vi "Reset Pin Names.vi"(0 "Display State In":T1, 7 "Connector":string="roboRIO 10 Bank Connector DIO", 9 "Container State":T2, 11 "error in (no error)":errorcluster) -> (4 "Display State Out":T1, 15 "error out":errorcluster)   [LabVIEW 2021, in "roboRIO 10 Bank.xctl"]
uses:
  <vilib>/myRIO/Common/Instrument Driver Framework/Utilities/xctls/roboRIO 10 Bank/roboRIO 10 Bank.xctl
  <vilib>/_xctls/Container State.ctl
  <vilib>/myRIO/Common/Instrument Driver Framework/Utilities/xctls/roboRIO 10 Bank/State.ctl
  <vilib>/myRIO/Common/Instrument Driver Framework/Utilities/xctls/utilities/vis/roboRIO Read Default State.vi
  <vilib>/_xctls/XControlSupport.lvlib
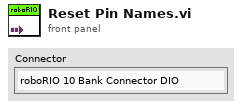
[diagram p1: front panel]
types:
  T1 = typedef "roboRIO 10 Bank.xctl/State.ctl" = cluster{"Pin Disabled?":enum8{"Enabled", "Disabled", "Disabled and Grayed Out"}[], "Pin Name":string[], "Pin ID":string[], "Connector Name":string, "Row Name 1":string, "Row Name 2":string}
  T2 = typedef "XControlSupport.lvlib/Container State.ctl" = cluster{"Indicator?":bool, "Run Mode?":bool, " Refnum":refnum<vi>}
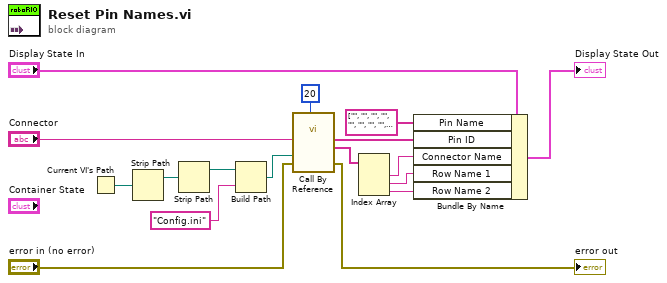
[diagram p0: block diagram]
diagram:
  n1 = Current VI's Path() -> (path=w16:path)
  n2 = Strip Path(path=w16) -> (stripped path=w15:path)  [unwired: 1 out]
  n3 = Strip Path(path=w15) -> (stripped path=w14:path)  [unwired: 1 out]
  n4 = Build Path(base path=w14, name or relative path="Config.ini") -> (appended path=w12:path)
  n5 = call-by-ref "?"("Size"=20, "error in"="error in (no error)", "Path"=w12, "Connector"="Connector") -> ("error out"=→"error out":errorcluster, "Default Connector Info"=w8:string[], "Default Pins Num"=w9:string[])  [unwired: 7 in, 2 out]
  n6 = Index Array(array=w8) -> (element #1=w7:string, element #2=w6:string, element #3=w5:string)  [unwired: 3 in]
  n7 = Bundle By Name(cluster="Display State In", "Pin Name"=string[] ["", "", "", "", "", "", "", "", "", "", "", "", "", "", "", "", "", "", "", ""] ("Pin Alias"), "Pin ID"=w9, "Connector Name"=w7, "Row Name 1"=w6, "Row Name 2"=w5) -> (→"Display State Out":T1)
